vi "NR Configure ACP.vi"(0 "RFmx Handle In":refnum<k21>, 1 "Selector String":string, 5 "NR ACP Configuration":T1={"Number of UTRA Offsets"=2, "Number of EUTRA Offsets"=1, "Number of NR Offsets"=1, "Number of ENDC Offsets"=0, "Measurement Method"=0, "Noise Compensation Enabled"=0, "Sweep Time Auto"=1, "Sweep Time Interval (s)"=0.001, "Averaging Enabled"=0, "Averaging Count"=10, "Averaging Type"=0} {"Measurement Method" items=["Normal", "Dynamic Range", "Sequential FFT"]; "Noise Compensation Enabled" items=["False", "True"]; "Sweep Time Auto" items=["False", "True"]; "Averaging Type" items=["RMS", "Log", "Scalar", "Max", "Min"]; "Averaging Enabled" items=["False", "True"]}, 11 "error in (no error)":errorcluster) -> (4 "RFmx Handle Out":refnum<k21>, 15 "error out":errorcluster)   [LabVIEW 2019, in "RFmxNR.lvlib"]
doc: "Configures common settings for the ACP measurement and selects the measurement."
uses:
  RFmxNR.lvlib
  Typedefs/NR ACP Configuration.ctl
  <vilib>/RFmx/NR/mx/RFmxNR.llb/RFmxNR Select Measurement (Single).vi
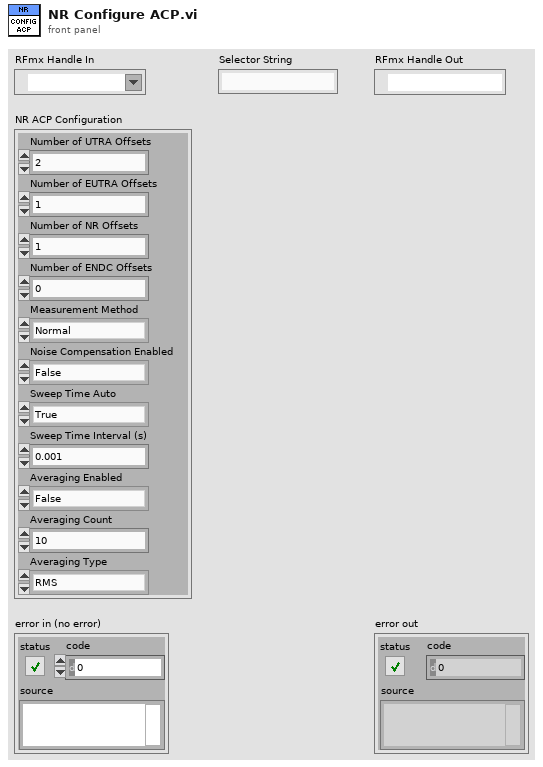
[diagram p1: front panel]
types:
  T1 = typedef "RFmxNR.lvlib/NR ACP Configuration.ctl" = cluster{"Number of UTRA Offsets":i32, "Number of EUTRA Offsets":i32, "Number of NR Offsets":i32, "Number of ENDC Offsets":i32, "Measurement Method":i32, "Noise Compensation Enabled":i32, "Sweep Time Auto":i32, "Sweep Time Interval (s)":dbl, "Averaging Enabled":i32, "Averaging Count":i32, "Averaging Type":i32}
  T2 = enum16{"ModAcc", "SEM", "ACP", "CHP", "OBW", "PVT"}
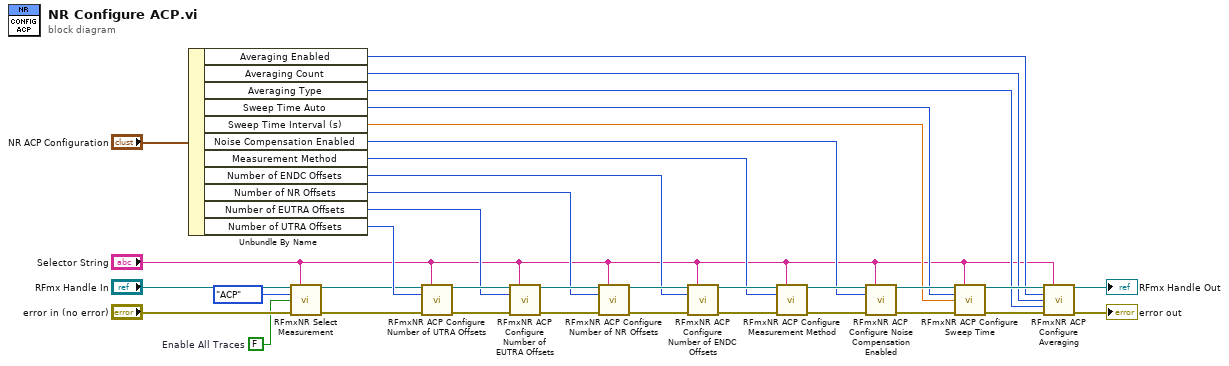
[diagram p0: block diagram]
diagram:
  w1 = FALSE  # Enable All Traces
  n1 = Unbundle By Name("NR ACP Configuration") -> ("Averaging Enabled"=w8:i32, "Averaging Count"=w7:i32, "Averaging Type"=w6:i32, "Sweep Time Auto"=w10:i32, "Sweep Time Interval (s)"=w9:dbl, "Noise Compensation Enabled"=w11:i32, "Measurement Method"=w12:i32, "Number of ENDC Offsets"=w13:i32, "Number of NR Offsets"=w14:i32, "Number of EUTRA Offsets"=w15:i32, "Number of UTRA Offsets"=w16:i32)
  n2 = call-poly <vilib>:"RFmxNR Select Measurement.vi"("Instrument Handle In"="RFmx Handle In", "Selector String"="Selector String", "Measurement"=T2."ACP", "Enable All Traces"=w1, "error in (no error)"="error in (no error)") -> ("Instrument Handle Out"=w4:refnum<k21>, "error out"=w27:errorcluster)  [unwired: 9 in]
  n3 = call <vilib>:"RFmxNR ACP Configure Number of UTRA Offsets.vi"("Instrument Handle In"=w4, "Selector String"="Selector String", "Number of UTRA Offsets"=w16, "error in (no error)"=w27) -> ("Instrument Handle Out"=w25:refnum<k21>, "error out"=w35:errorcluster)  [unwired: 10 in]
  n4 = call <vilib>:"RFmxNR ACP Configure Number of EUTRA Offsets.vi"("Instrument Handle In"=w25, "Selector String"="Selector String", "Number of EUTRA Offsets"=w15, "error in (no error)"=w35) -> ("Instrument Handle Out"=w24:refnum<k21>, "error out"=w34:errorcluster)  [unwired: 10 in]
  n5 = call <vilib>:"RFmxNR ACP Configure Number of NR Offsets.vi"("Instrument Handle In"=w24, "Selector String"="Selector String", "Number of NR Offsets"=w14, "error in (no error)"=w34) -> ("Instrument Handle Out"=w23:refnum<k21>, "error out"=w33:errorcluster)  [unwired: 10 in]
  n6 = call <vilib>:"RFmxNR ACP Configure Number of ENDC Offsets.vi"("Instrument Handle In"=w23, "Selector String"="Selector String", "Number of ENDC Offsets"=w13, "error in (no error)"=w33) -> ("Instrument Handle Out"=w22:refnum<k21>, "error out"=w32:errorcluster)  [unwired: 10 in]
  n7 = call <vilib>:"RFmxNR ACP Configure Measurement Method.vi"("Instrument Handle In"=w22, "Selector String"="Selector String", "Measurement Method"=w12, "error in (no error)"=w32) -> ("Instrument Handle Out"=w21:refnum<k21>, "error out"=w31:errorcluster)  [unwired: 10 in]
  n8 = call <vilib>:"RFmxNR ACP Configure Noise Compensation Enabled.vi"("Instrument Handle In"=w21, "Selector String"="Selector String", "Noise Compensation Enabled"=w11, "error in (no error)"=w31) -> ("Instrument Handle Out"=w20:refnum<k21>, "error out"=w30:errorcluster)  [unwired: 10 in]
  n9 = call <vilib>:"RFmxNR ACP Configure Sweep Time.vi"("Instrument Handle In"=w20, "Selector String"="Selector String", "Sweep Time Auto"=w10, "Sweep Time Interval (s)"=w9, "error in (no error)"=w30) -> ("Instrument Handle Out"=w19:refnum<k21>, "error out"=w29:errorcluster)  [unwired: 9 in]
  n10 = call <vilib>:"RFmxNR ACP Configure Averaging.vi"("Instrument Handle In"=w19, "Selector String"="Selector String", "Averaging Enabled"=w8, "Averaging Count"=w7, "Averaging Type"=w6, "error in (no error)"=w29) -> ("Instrument Handle Out"=→"RFmx Handle Out":refnum<k21>, "error out"=→"error out":errorcluster)  [unwired: 8 in]
